vi "Remove points in historam by sd.vi"() -> ()   [LabVIEW 2021]
uses:
  <vilib>/Utility/file.llb/Read Delimited Spreadsheet (DBL).vi
  <vilib>/Utility/file.llb/Write Delimited Spreadsheet (DBL).vi
  <vilib>/Analysis/NI_AALBase.lvlib
panel:
  in  "Name extend":string="_reduced"
  in  "devriation":dbl=3.0 format="%#_13g"
  out "Progress %":dbl=98.36065573770492
  in  "book number":i32=475
  in  "file path (dialog if empty)":path=path "C:/Users/gyue/Box Sync/Guang Yue/data/Contour plot"
  # "Remove data points outside average+sd range"
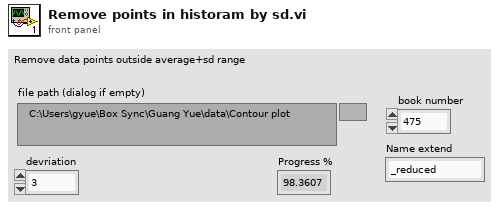
[diagram p1: front panel]
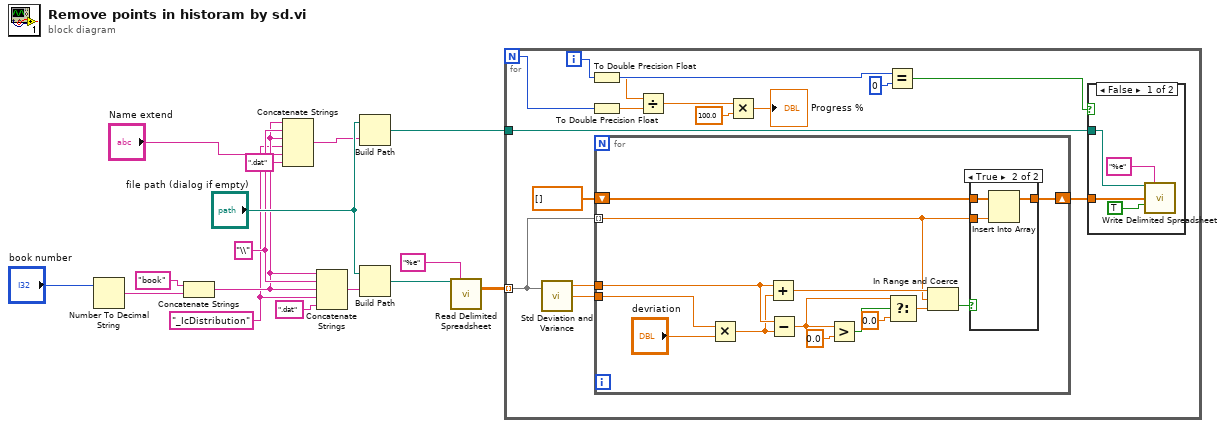
[diagram p0: block diagram]
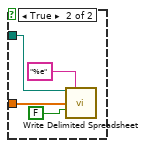
[diagram p2: hidden frame]
diagram:
  w5 = "_IcDistribution" ("string")
  w7 = "\\" ("string")
  n1 = Number To Decimal String(number="book number") -> (decimal integer string=w14:string)  [unwired: 1 in]
  n2 = Concatenate Strings("book" ("string"), w14) -> (w6:string)
  n3 = Concatenate Strings(w6, w7, w6, w5, "Name extend", ".dat" ("string")) -> (w3:string)
  n4 = Concatenate Strings(w6, w7, w6, w5, ".dat" ("string")) -> (w15:string)
  n5 = Build Path(base path="file path (dialog if empty)", name or relative path=w3) -> (appended path=w2:path)
  n6 = Build Path(base path="file path (dialog if empty)", name or relative path=w15) -> (appended path=w16:path)
  n7 = call-poly <vilib>:"Read Delimited Spreadsheet.vi"("file path (dialog if empty)"=w16, "format (%.3f)"="%e") -> ("all rows"=w10:dbl[][])  [unwired: 8 in, 5 out]
  n8 = for {
    N -> [w31]
    tunnel: w10 -> [w27] mode=indexing
    tunnel: w2 -> [w18]
    i -> [w23]
    n9 = call <vilib>:"Std Deviation and Variance.vi"("X"=w27) -> ("mean"=w26:dbl, "standard deviation"=w25:dbl)  [unwired: 1 in, 1 out]
    n10 = To Double Precision Float(number=w23) -> (double precision float=w20:dbl)
    n11 = To Double Precision Float(number=w31) -> (double precision float=w19:dbl)
    n12 = for {
      tunnel: w27 -> [w47] mode=indexing
      tunnel: w26 -> [w50]
      tunnel: w25 -> [w53]
      shift-right: [w45] -> w17
      shift-left: dbl[] [] -> [w46]
      n13 = Multiply(x=w53, y="devriation") -> (x*y=w49:dbl)
      n14 = Add(x=w50, y=w49) -> (x+y=w51:dbl)
      n15 = Subtract(x=w50, y=w49) -> (x-y=w42:dbl)
      n16 = Greater?(x=w42, y=0.0) -> (0:w43:bool)
      n17 = Select(t=w42, s=w43, f=0.0) -> (s? t:f=w40:dbl)
      n18 = In Range and Coerce(upper limit=w51, x=w47, lower limit=w40) -> (In Range?=w48:bool)  [unwired: 1 out]
      n19 = case shown="True" w48 {
        tunnel: w47 -> [_ w56]
        tunnel: w46 -> [w54 w57]
        tunnel: [w54 w55] -> w45
        frame False {
        }
        frame True {
          n20 = Insert Into Array(array=w57, new element=w56) -> (w55:dbl[])  [unwired: 1 in]
        }
      }
    }
    n21 = Divide(x=w20, y=w19) -> (x/y=w30:dbl)
    n22 = Multiply(x=w30, y=100.0) -> (x*y=→"Progress %":dbl)
    n23 = Equal?(x=w23, y=0) -> (x = y?=w21:bool)
    n24 = case shown="False" w21 {
      tunnel: w18 -> [w32 w39]
      tunnel: w17 -> [w33 w36]
      frame False {
        n25 = call-poly <vilib>:"Write Delimited Spreadsheet.vi"("file path (dialog if empty)"=w32, "format (%.3f)"="%e" ("format (%d)"), "1D data"=w33, "append to file? (new file:F)"=TRUE) -> ()  [unwired: 10 in, 2 out]
      }
      frame True {
        n26 = call-poly <vilib>:"Write Delimited Spreadsheet.vi"("file path (dialog if empty)"=w39, "format (%.3f)"="%e" ("format (%d)"), "1D data"=w36, "append to file? (new file:F)"=FALSE) -> ()  [unwired: 10 in, 2 out]
      }
    }
  }
